vi "Ini_Read_LoadDir.vi"(8 "error in (no error)":errorcluster) -> (0 "error out":errorcluster caption="sortie d'erreur", 3 "Path":path)   [LabVIEW 2020]
doc: "This VI reads the parameter \"LoadDir\" from the PIL.ini file, located at the main directory."
uses:
  <vilib>/Utility/config.llb/Read Key (Path).vi
  <vilib>/Utility/config.llb/NI_LVConfig.lvlib
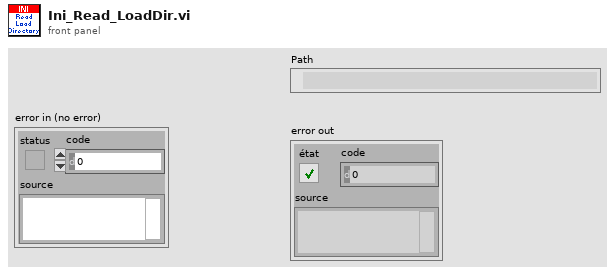
[diagram p1: front panel]
types:
  T1 = typedef "NI_LVConfig.lvlib/Config Data RefNum.ctl" = refnum<k1>
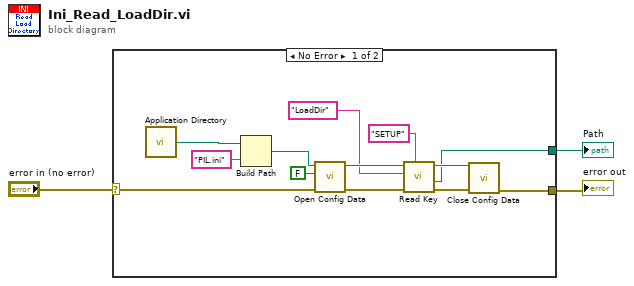
[diagram p0: block diagram]
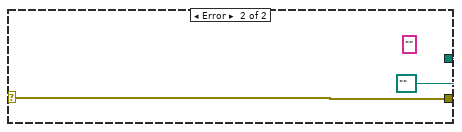
[diagram p2: hidden frame]
diagram:
  n1 = case shown="No Error" "error in (no error)" {
    selector: "error in (no error)" -> [w6 w18]
    tunnel: [w5 w18] -> w2
    tunnel: [w4 path "" ("Data Path")] -> w1
    frame No Error {
      n2 = call <vilib>:"Application Directory.vi"() -> ("Application Directory"=w16:path)
      n3 = Build Path(base path=w16, name or relative path="PIL.ini" ("nom ou chemin relatif")) -> (appended path=w15:path)
      n4 = call <vilib>:"Open Config Data.vi"("error in (no error)"=w6, "create file if necessary (T)"=FALSE, "configuration file path"=w15) -> ("error out"=w12:errorcluster, "refnum"=w11:T1)  [unwired: 6 in, 1 out]
      n5 = call-poly <vilib>:"Read Key.vi"("section"="SETUP", "error in (no error)"=w12, "key"="LoadDir", "refnum"=w11) -> ("error out"=w14:errorcluster, "value"=w4:path, "refnum out"=w13:T1)  [unwired: 4 in, 1 out]
      n6 = call <vilib>:"Close Config Data.vi"("error in (no error)"=w14, "refnum"=w13) -> ("error out"=w5:errorcluster)  [unwired: 8 in, 1 out]
    }
    frame Error {
      (unwired) "" ("XML File Filter")
    }
  }
  "error out" <- w2
  "Path" <- w1
